vi "Serial Read Write UWB.vi"(0 "Transmit":refnum<k21>="Port8/DIO0", 1 "Receive":refnum<k21>="Port8/DIOCTL", 2 "baud rate (115200)":u32=9600, 3 "data bits (8)":i32=8 min=5 max=8 step=1, 7 "stop bits (10: 1 bit)":u16(ring)=10 items=["1.0"=10, "1.5"=15, "2.0"=20], 11 "Invert Polarity?":bool) -> ()   [LabVIEW 2016]
uses:
  <vilib>/rvi/Emulation/niFpgaGetClockAttributes.vi
  <vilib>/rvi/Emulation/niFpgaSctlEmulationGetInTimedLoop.vi
  <vilib>/rvi/Emulation/niFpgaEmulationReportErrorSimple.vi
  <vilib>/rvi/eio/common/nirviEmuTemplateMethod_errors.vi
  <vilib>/rvi/Emulation/niFpgaProcessEmulError.vi
  <vilib>/rvi/DataTransferAndStorage/Container/Common/niFpgaContainerExecOnDevCompGetState.vi
  <vilib>/rvi/Emulation/niFpgaEmulationIsFPGAContextNoSignature.vi
  <vilib>/rvi/errors/niFpgaSetErrorForExecOnDevCompSimple.vi
  <vilib>/rvi/eio/common/nirviEmuReportErrorAndStop.vi
  <vilib>/rvi/DataTransferAndStorage/Container/Common/niFpgaContainerGetUniqueNameForEmu.vi
  <vilib>/rvi/FIFO/Fifo_Resource/nirvififoEmulationSetSize.vi
  <vilib>/rvi/FIFO/Fifo_Resource/nirviFifoEmulationQueueMgr.vi
  <instcachedir>/0/nirviFifoEmulationQueueMgr_E5CAEC123FF24DC58D834DCA3CDAA9B5.lvgen/nirviFifoEmulationQueueMgr_E5CAEC123FF24DC58D834DCA3CDAA9B5_000.vi
  <vilib>/rvi/FIFO/Fifo_Resource/nirvififoEmulationDetermineInputValidOut.vi
  <vilib>/rvi/FIFO/Fifo_Resource/nirvififoEmulationCreateLock.vi
  <vilib>/rvi/FIFO/Fifo_Resource/nirvififoEmulationObtainLock.vi
  <vilib>/rvi/FIFO/Fifo_Resource/nirvififoEmulationReleaseLock.vi
  <vilib>/rvi/occurrence/nirviWaitOnOccurrenceBase.vi
  <vilib>/rvi/errors/nirviReportUnexpectedCaseInternalError.vi
  <vilib>/rvi/errors/nirviReportUnexpectedCaseInternalError (U32).vi
  <vilib>/Utility/error.llb/Clear Errors.vi
  <vilib>/rvi/interface/RandomDataEmulation/niFpgaRandomDataHandleErrors.vi
  <vilib>/rvi/Emulation/niFpgaCriticalErrorInLSC.vi
  Instance           1 27Saved   LV FPGA Serial Read .vi
  Instance           2 27Saved   LV FPGA Serial Read .vi
  Instance           6 27Saved   LV FPGA Serial Read .vi
  <vilib>/eio/EIOMethodNode/EIOMethodNode.xnode
  <vilib>/rvi/DataTransferAndStorage/Container/XNode/niFpgaContainer.xnode
  <vilib>/rvi/FIFO/Fifo_Resource/niFpgaFifoEmulationRefIn.vi
  <vilib>/eio/EIONode/EIONode.xnode
panel:
  out "Read: Transmission Error":bool
  in  "stop":bool
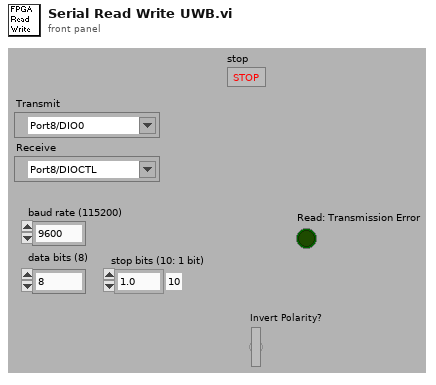
[diagram p1: front panel]
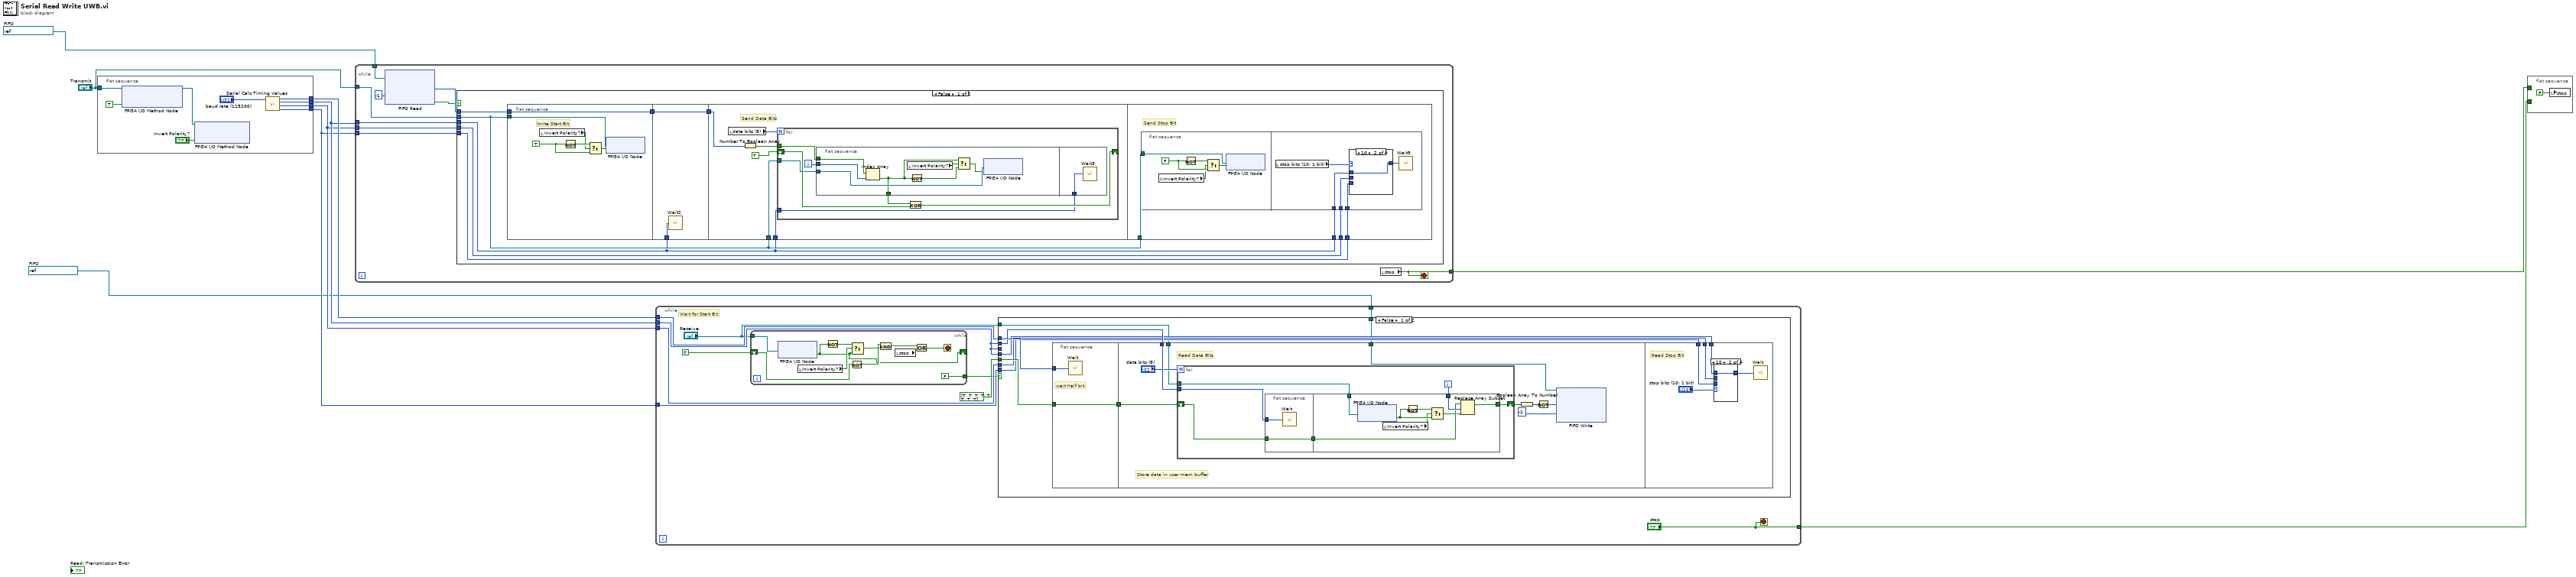
[diagram p0: block diagram]
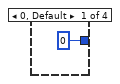
[diagram p2: hidden frame]
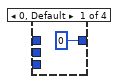
[diagram p6: hidden frame]
diagram:
  w1 = refnum<k21> "Read FIFO UWB"  # FIFO
  w2 = refnum<k21> "Write FIFO UWB"  # FIFO
  n1 = flat-sequence {
    tunnel: [w13] -> w8
    tunnel: [w14] -> w9
    tunnel: [w12] -> w7
    tunnel: [w11] -> w6
    tunnel: "Transmit" -> [w17]
    frame #0 {
      n2 = xnode "FPGA I/O Method Node"("FPGA I/O In"=w17, "Enable"=TRUE ("Digital Enable")) -> ("FPGA I/O Out"=w16:refnum<k21>)
      n3 = xnode "FPGA I/O Method Node"("FPGA I/O In"=w16, "Data"="Invert Polarity?") -> ()  [unwired: 1 out]
      n4 = call "Serial Calc Timing Values.vi"("baud rate (1000000)"="baud rate (115200)") -> ("Two Bit"=w11:u32, "One and Half Bit"=w12:u32, "One Bit"=w13:u32, "Half Bit"=w14:u32)  [unwired: 3 in]
    }
  }
  n5 = while {
    tunnel: w6 -> [w27]
    tunnel: w7 -> [w26]
    tunnel: w8 -> [w25]
    tunnel: "Transmit" -> [w24]
    tunnel: [w21] -> w3
    tunnel: w2 -> [w19]
    stop <- w21 stop-if-true
    n6 = xnode ("FIFO Read")("Timeout"=-1, "FIFO In"=w19) -> ("Element"=w23:u8, "Timed Out?"=w22:bool)  [unwired: 1 out]
    n7 = case shown="False" w22 {
      tunnel: w27 -> [w32 _]
      tunnel: w26 -> [w31 _]
      tunnel: w25 -> [w28 _]
      tunnel: w24 -> [w30 _]
      tunnel: w23 -> [w29 _]
      frame False {
        n8 = flat-sequence {
          tunnel: w30 -> [w40]
          tunnel: w29 -> [w35]
          tunnel: [w35] -> w34
          tunnel: w28 -> [w42]
          tunnel: [w41] -> w33
          tunnel: w34 -> [w41]
          tunnel: w33 -> [w43]
          tunnel: w30 -> [w44]
          tunnel: w28 -> [w48]
          tunnel: w28 -> [w67]
          tunnel: w31 -> [w66]
          tunnel: w32 -> [w65]
          tunnel: w30 -> [w64]
          frame #0 {
            w38 = TRUE
            # "Write Start Bit"
            n9 = local read "Invert Polarity?"() -> (w37:bool)
            n10 = Not(x=w38) -> (.not. x?=w39:bool)
            n11 = Select(t=w39, s=w37, f=w38) -> (s? t:f=w36:bool)
            n12 = xnode "FPGA I/O Node"("I/O Item"=w36, "FPGA I/O In"=w40) -> ()  [unwired: 1 out]
          }
          frame #1 {
            n13 = call "Wait2"("Count(Ticks)"=w42) -> ()  [unwired: 1 out]
          }
          frame #2 {
            # "Send Data Bits"
            n14 = local read "data bits (8)"() -> (w45:i32)
            n15 = Number To Boolean Array(number=w43) -> (Boolean array=w46:bool[])
            n16 = for {
              N: w45 -> [_]
              tunnel: w48 -> [w52]
              shift-right: [w55] -> _
              shift-left: TRUE -> [w54]
              tunnel: w46 -> [w51]
              tunnel: w44 -> [w49]
              i -> [w53]
              n17 = flat-sequence {
                tunnel: w53 -> [w62]
                tunnel: w51 -> [w61]
                tunnel: [w56] -> w50
                tunnel: w49 -> [w60]
                tunnel: w52 -> [w63]
                frame #0 {
                  n18 = Index Array(array=w61, index=w62) -> (element=w56:bool)
                  n19 = local read "Invert Polarity?"() -> (w58:bool)
                  n20 = Not(x=w56) -> (.not. x?=w59:bool)
                  n21 = Select(t=w56, s=w58, f=w59) -> (s? t:f=w57:bool)
                  n22 = xnode "FPGA I/O Node"("I/O Item"=w57, "FPGA I/O In"=w60) -> ()  [unwired: 1 out]
                }
                frame #1 {
                  n23 = call "Wait3"("Count(Ticks)"=w63) -> ()  [unwired: 1 out]
                }
              }
              n24 = Exclusive Or(1:w54, 2:w50) -> (0:w55:bool)
            }
          }
          frame #3 {
            # "Send Stop Bit"
            n25 = flat-sequence {
              tunnel: w64 -> [w72]
              tunnel: w65 -> [w75]
              tunnel: w66 -> [w76]
              tunnel: w67 -> [w77]
              frame #0 {
                w70 = FALSE
                n26 = local read "Invert Polarity?"() -> (w69:bool)
                n27 = Not(x=w70) -> (.not. x?=w71:bool)
                n28 = Select(t=w71, s=w69, f=w70) -> (s? t:f=w68:bool)
                n29 = xnode "FPGA I/O Node"("I/O Item"=w68, "FPGA I/O In"=w72) -> ()  [unwired: 1 out]
              }
              frame #1 {
                n30 = local read "stop bits (10: 1 bit)"() -> (w73:u16)
                n31 = case shown="10" w73 {
                  tunnel: w77 -> [_ w79 _ _]
                  tunnel: w76 -> [_ _ w80 _]
                  tunnel: w75 -> [_ _ _ w81]
                  tunnel: [u32 0 ("One Bit") w79 w80 w81] -> w74
                  frame 0, Default {
                  }
                  frame 10 {
                  }
                  frame 15 {
                  }
                  frame 20 {
                  }
                }
                n32 = call "Wait5"("Count(Ticks)"=w74) -> ()  [unwired: 1 out]
              }
            }
          }
        }
      }
      frame True {
      }
    }
    n33 = local read "stop"() -> (w21:bool)
  }
  n34 = while {
    tunnel: w6 -> [w90]
    tunnel: w7 -> [w89]
    tunnel: w8 -> [w88]
    tunnel: w9 -> [w87]
    tunnel: ["stop"] -> w4
    tunnel: w1 -> [w82]
    stop <- "stop" stop-if-true
    # "Wait for Start Bit"
    n35 = while {
      tunnel: [FALSE] -> w86
      shift-right: [w92] -> _
      shift-left: TRUE -> [w101]
      tunnel: "Receive" -> [w96]
      stop <- w97 stop-if-true
      n36 = xnode "FPGA I/O Node"("FPGA I/O In"=w96) -> ("I/O Item"=w92:bool)  [unwired: 1 out]
      n37 = local read "Invert Polarity?"() -> (w94:bool)
      n38 = Not(x=w92) -> (.not. x?=w95:bool)
      n39 = Not(x=w101) -> (.not. x?=w100:bool)
      n40 = Select(t=w95, s=w94, f=w92) -> (s? t:f=w93:bool)
      n41 = And(x=w100, y=w93) -> (x .and. y?=w98:bool)
      n42 = local read "stop"() -> (w99:bool)
      n43 = Or(x=w98, y=w99) -> (x .or. y?=w97:bool)
    }
    n44 = case shown="False" w86 {
      tunnel: bool[] [TRUE, TRUE, TRUE, TRUE, TRUE, TRUE, TRUE, TRUE] -> [w111 _]
      tunnel: w87 -> [w110 _]
      tunnel: w88 -> [w109 _]
      tunnel: w88 -> [_ _]
      tunnel: w88 -> [w108 _]
      tunnel: w89 -> [w107 _]
      tunnel: w90 -> [w106 _]
      tunnel: "Receive" -> [w105 _]
      tunnel: w82 -> [w103 _]
      frame False {
        n45 = flat-sequence {
          tunnel: [w113] -> w104
          tunnel: w110 -> [w112]
          tunnel: w111 -> [w113]
          tunnel: w104 -> [w122]
          tunnel: w109 -> [w121]
          tunnel: w105 -> [w117]
          tunnel: w103 -> [w114]
          tunnel: w106 -> [w140]
          tunnel: w107 -> [w141]
          tunnel: w108 -> [w142]
          frame #0 {
            # "wait half bit"
            n46 = call "Wait"("Count(Ticks)"=w112) -> ()  [unwired: 1 out]
          }
          frame #1 {
            # "Store data in user mem buffer"
            # "Read Data Bits"
            n47 = for {
              N: "data bits (8)" -> [_]
              shift-right: [w126] -> w120
              shift-left: w122 -> [w128]
              tunnel: w121 -> [w127]
              tunnel: w117 -> [w124]
              i -> [w125]
              n48 = flat-sequence {
                tunnel: w128 -> [w130]
                tunnel: [w130] -> w123
                tunnel: w127 -> [w129]
                tunnel: [w138] -> w126
                tunnel: w124 -> [w134]
                tunnel: w125 -> [w136]
                tunnel: w123 -> [w135]
                frame #0 {
                  n49 = call "Wait"("Count(Ticks)"=w129) -> ()  [unwired: 1 out]
                }
                frame #1 {
                  n50 = xnode "FPGA I/O Node"("FPGA I/O In"=w134) -> ("I/O Item"=w137:bool)  [unwired: 1 out]
                  n51 = local read "Invert Polarity?"() -> (w133:bool)
                  n52 = Not(x=w137) -> (.not. x?=w132:bool)
                  n53 = Select(t=w132, s=w133, f=w137) -> (s? t:f=w131:bool)
                  n54 = Replace Array Subset(array=w135, new element=w131, index=w136) -> (w138:bool[])
                }
              }
            }
            n55 = Boolean Array To Number(Boolean array=w120) -> (number=w119:u8)
            n56 = Not(x=w119) -> (.not. x?=w116:u8)
            n57 = xnode ("FIFO Write")("Element"=w116, "Timeout"=-1, "FIFO In"=w114) -> ()  [unwired: 2 out]
          }
          frame #2 {
            # "Read Stop Bit"
            n58 = case shown="10" "stop bits (10: 1 bit)" {
              tunnel: w142 -> [_ w145 _ _]
              tunnel: w141 -> [_ _ w146 _]
              tunnel: w140 -> [_ _ _ w147]
              tunnel: [u32 0 ("One Bit") w145 w146 w147] -> w139
              frame 0, Default {
              }
              frame 10 {
              }
              frame 15 {
              }
              frame 20 {
              }
            }
            n59 = call "Wait"("Count(Ticks)"=w139) -> ()  [unwired: 1 out]
          }
        }
      }
      frame True {
      }
    }
  }
  n60 = flat-sequence {
    tunnel: w4 -> [_]
    tunnel: w3 -> [_]
    frame #0 {
      n61 = local write "stop"(FALSE ("stop")) -> ()
    }
  }
